vi "ueye allocate image memory.vi"(0 "Camera reference in":refnum<k24>, 5 "Error In":errorcluster) -> (12 "Camera reference out":refnum<k24>, 14 "Bits/Pixel 2":i32=8, 15 "Width":i32, 16 "Serial Number":string, 17 "Height":i32, 19 "Error Out":errorcluster)   [LabVIEW 2022 SP3, in "Vision.lvlib"]
uses:
  Vision.lvlib
  C:/Users/Caleb/Desktop/nebraska-silicon-lab/pixel-gantry-control/Gantry/Shared Components/bin/uEyeDotNet.dll
  bin/uEyeDotNet.dll
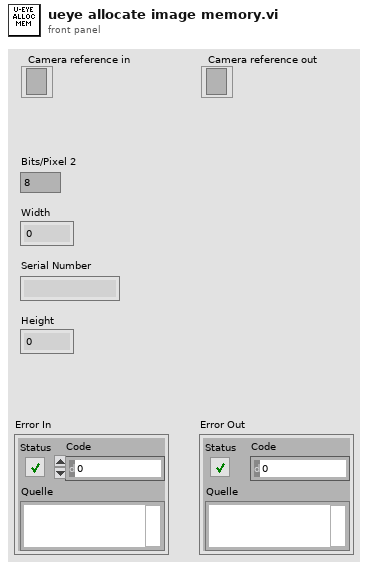
[diagram p1: front panel]
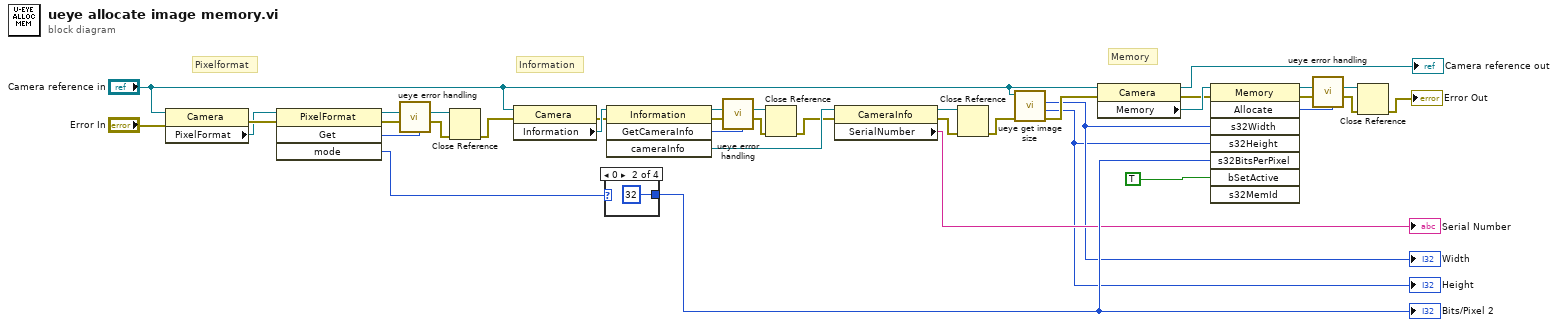
[diagram p0: block diagram]
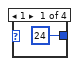
[diagram p2: hidden frame]
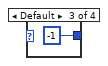
[diagram p3: hidden frame]
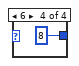
[diagram p4: hidden frame]
diagram:
  # "Information"
  # "Memory"
  # "Pixelformat"
  n1 = property class="Camera"(reference="Camera reference in", error in="Error In") -> (error out=w31:errorcluster, "PixelFormat"=w30:refnum<k24>)  [unwired: 1 out]
  n2 = invoke class="PixelFormat" method="Get"(reference=w30, error in=w31) -> (reference out=w13:refnum<k24>, error out=w23:errorcluster, "Get"=w18:i32, "mode"=w27:i32)  [unwired: 2 in]
  n3 = call "ueye error handling.vi"("Error Code"=w18, "reference in"=w13, "Error In"=w23) -> ("Error Out"=w12:errorcluster)  [unwired: 8 in]
  n4 = Close Reference(reference=w13, error in (no error)=w12) -> (error out=w11:errorcluster)
  n5 = property class="Camera"(reference="Camera reference in", error in=w11) -> (error out=w28:errorcluster, "Information"=w29:refnum<k24>)  [unwired: 1 out]
  n6 = case shown="0" w27 {
    tunnel: [24 32 -1 8] -> w35
    frame 1 {
    }
    frame 0 {
    }
    frame Default {
    }
    frame 6 {
    }
  }
  "Bits/Pixel 2" <- w35
  n7 = invoke class="Information" method="GetCameraInfo"(reference=w29, error in=w28) -> (reference out=w9:refnum<k24>, error out=w17:errorcluster, "GetCameraInfo"=w16:i32, "cameraInfo"=w25:refnum<k24>)  [unwired: 2 in]
  n8 = call "ueye error handling.vi"("Error Code"=w16, "reference in"=w9, "Error In"=w17) -> ("Error Out"=w10:errorcluster)  [unwired: 8 in]
  n9 = Close Reference(reference=w9, error in (no error)=w10) -> (error out=w8:errorcluster)
  n10 = property class="CameraInfo"(reference=w25, error in=w8) -> (reference out=w7:refnum<k24>, error out=w6:errorcluster, "SerialNumber"=→"Serial Number":string)
  n11 = Close Reference(reference=w7, error in (no error)=w6) -> (error out=w5:errorcluster)
  n12 = call "ueye get image size.vi"("Error In"=w5, "Camera reference in"="Camera reference in") -> ("Error Out"=w22:errorcluster, "Height"=w19:i32, "Width"=w20:i32)  [unwired: 6 in, 1 out]
  "Height" <- w19
  "Width" <- w20
  n13 = property class="Camera"(reference="Camera reference in", error in=w22) -> (reference out=→"Camera reference out":refnum<k24>, error out=w32:errorcluster, "Memory"=w33:refnum<k24>)
  n14 = invoke class="Memory" method="Allocate"(reference=w33, error in=w32, "s32Width"=w20, "s32Height"=w19, "s32BitsPerPixel"=w35, "bSetActive"=TRUE) -> (reference out=w4:refnum<k24>, error out=w15:errorcluster, "Allocate"=w14:i32)  [unwired: 2 in, 5 out]
  n15 = call "ueye error handling.vi"("Error Code"=w14, "reference in"=w4, "Error In"=w15) -> ("Error Out"=w3:errorcluster)  [unwired: 8 in]
  n16 = Close Reference(reference=w4, error in (no error)=w3) -> (error out=→"Error Out":errorcluster)
